vi "Day 9-Find Low Points.vi"(11 "Array in":i32[][](array[numeric])) -> (2 "Low Point Coordinates":i32[][](array[numeric]), 3 "Low Point Values":i32[](array[numeric]))   [LabVIEW 2021]
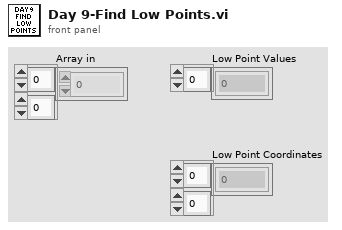
[diagram p1: front panel]
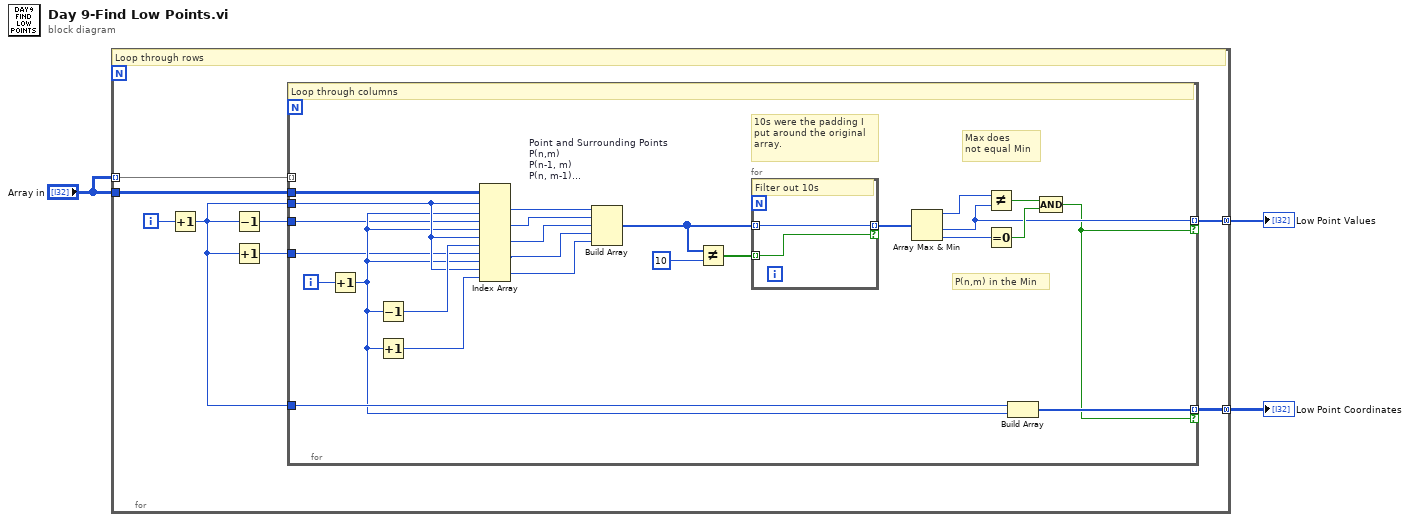
[diagram p0: block diagram]
diagram:
  n1 = for {
    tunnel: [w11] -> w3 mode=concatenating
    tunnel: "Array in" -> [w10] mode=indexing
    tunnel: "Array in" -> [w8]
    tunnel: [w4] -> w2 mode=concatenating
    i -> [w9]
    # "Loop through rows"
    n2 = Increment(x=w9) -> (x+1=w6:i32)
    n3 = Decrement(x=w6) -> (x-1=w7:i32)
    n4 = Increment(x=w6) -> (x+1=w5:i32)
    n5 = for {
      tunnel: w8 -> [w36]
      tunnel: w6 -> [w28]
      tunnel: w6 -> [w26]
      tunnel: [w25] -> w11 mode=indexing if=w12
      tunnel: w10 -> [_] mode=indexing
      tunnel: w7 -> [w15]
      tunnel: w5 -> [w14]
      tunnel: [w13] -> w4 mode=indexing if=w12
      i -> [w20]
      # "Max does \nnot equal Min"
      # "P(n,m) in the Min"
      # "10s were the padding I put around the original array."
      # "Loop through columns"
      n6 = Increment(x=w20) -> (x+1=w19:i32)
      n7 = Decrement(x=w19) -> (x-1=w30:i32)
      n8 = Increment(x=w19) -> (x+1=w29:i32)
      n9 = Index Array(array=w36, index (row) #1=w28, index (col) #1=w19, index (row) #2=w15, index (col) #2=w19, index (row) #3=w28, index (col) #3=w30, index (row) #4=w14, index (col) #4=w19, index (row) #5=w28, index (col) #5=w29) -> (element #1=w27:i32, element #2=w35:i32, element #3=w34:i32, element #4=w33:i32, element #5=w32:i32)
      n10 = Build Array "Point and Surrounding Points\nP(n,m)\nP(n-1, m)\nP(n, m-1)\nP(n+1,m)\nP(n, m+1)"(w27, w35, w34, w33, w32) -> (w17:i32[])
      n11 = Not Equal?(x=w17, y=10) -> (x != y?=w16:bool[])
      n12 = for {
        tunnel: w17 -> [w38] mode=indexing
        tunnel: [w38] -> w21 mode=indexing if=w37
        tunnel: w16 -> [w37] mode=indexing
        # "Filter out 10s"
      }
      n13 = Array Max & Min(array=w21) -> (max value=w22:i32, min value=w13:i32, min index (indices)=w31:i32)  [unwired: 1 out]
      n14 = Not Equal?(x=w22, y=w13) -> (x != y?=w24:bool)
      n15 = Equal To 0?(x=w31) -> (x = 0?=w23:bool)
      n16 = Build Array(w26, w19) -> (w25:i32[])
      n17 = Compound Arithmetic op=AND(w24, w23) -> (w12:bool)
    }
  }
  "Low Point Coordinates" <- w3
  "Low Point Values" <- w2
